vi "DBLProblem.vi"() -> ()   [LabVIEW 2023]
panel:
  out "x+1":dbl
  out "double precision float":dbl format="%#_6f"
  out "number":dbl format="%#_6f"
  out "concatenated string":string
  in  "String 3":string
  in  "String 2":string
  in  "String":string
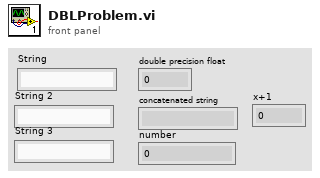
[diagram p1: front panel]
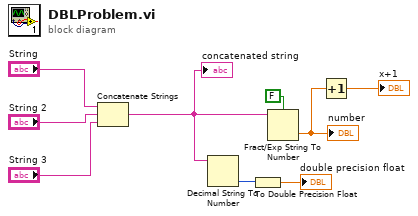
[diagram p0: block diagram]
diagram:
  n1 = Concatenate Strings("String", "String 2", "String 3") -> (w3:string)
  "concatenated string" <- w3
  n2 = Decimal String To Number(string=w3) -> (number=w5:i32)  [unwired: 2 in, 1 out]
  n3 = To Double Precision Float(number=w5) -> (double precision float=→"double precision float":dbl)
  n4 = Fract/Exp String To Number(use system decimal point (T)=FALSE, string=w3) -> (number=w2:dbl)  [unwired: 2 in, 1 out]
  "number" <- w2
  n5 = Increment(x=w2) -> (x+1=→"x+1":dbl)
